vi "Add Item to ListView by Text and ImageIndex.vi"(8 "error in (no error)":errorcluster caption="错误输入（无错误）", 9 "imageIndex":i32, 10 "text":string, 11 "ListViewClass 输入":refnum<class "ListViewClass.lvclass"> caption="DNL_LabVIEW Object in") -> (0 "error out":errorcluster caption="错误输出", 3 "ListViewClass 输出":refnum<class "ListViewClass.lvclass"> caption="DNL_LabVIEW Object out")   [LabVIEW 2012, in "ListViewClass.lvclass"]
uses:
  ListViewClass.lvclass
  ListViewClass.lvclass/ListViewClass.ctl
  System.Windows.Forms
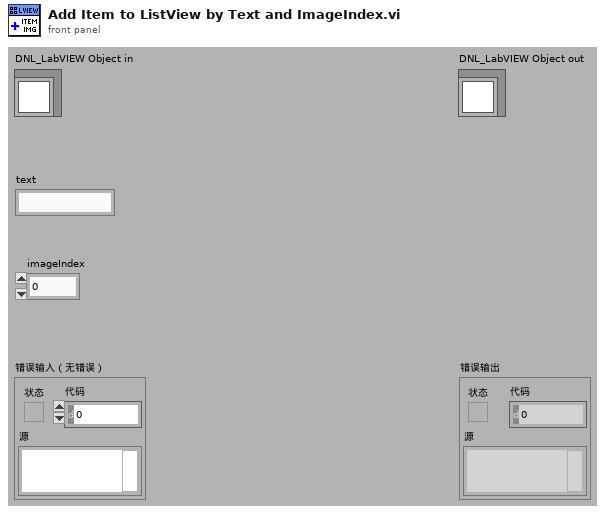
[diagram p1: front panel]
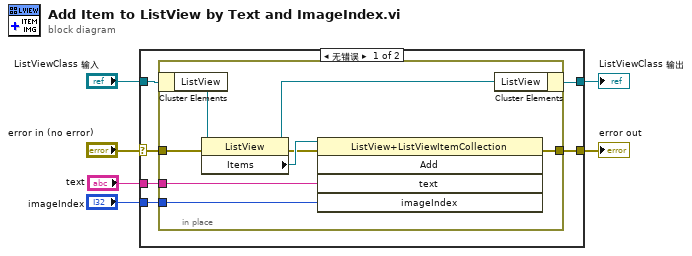
[diagram p0: block diagram]
diagram:
  n1 = case shown="无错误" "error in (no error)" {
    selector: "error in (no error)" -> [w11 w22]
    tunnel: [w9 w22] -> w5
    tunnel: [w10 w21] -> w3
    tunnel: "ListViewClass 输入" -> [w12 w21]
    tunnel: "text" -> [w8 _]
    tunnel: "imageIndex" -> [w7 _]
    frame No Error {
      n2 = in-place {
        in-place-border: w11 -> [w18]
        in-place-border: [w15] -> w9
        in-place-border: w8 -> [w14]
        in-place-border: w7 -> [w13]
        n3 = in-place-cluster #1(w12) -> ("ListView"=w20:refnum<k24>)
        n4 = property class="ListView"(reference=w20, error in=w18) -> (reference out=w16:refnum<k24>, error out=w17:errorcluster, "Items"=w19:refnum<k24>)
        n5 = invoke class="ListView+ListViewItemCollection" method="Add"(reference=w19, error in=w17, "text"=w14, "imageIndex"=w13) -> (error out=w15:errorcluster)  [unwired: 1 in, 4 out]
        n6 = in-place-cluster #1("ListView"=w16) -> (w10:refnum<class "ListViewClass.lvclass">)
      }
    }
    frame Error {
    }
  }
  "error out" <- w5
  "ListViewClass 输出" <- w3
